vi "mules_date2string.vi"(6 "date slash?":bool, 7 "time":timestamp, 8 "time colon?":bool, 9 "seconds?":bool, 10 "log_time":bool, 11 "now?":bool=TRUE) -> (1 "time_string":string, 2 "mm/dd/yyyy":string, 3 "date_time_string":string)   [LabVIEW 2013]
doc: "Da formato a los datos de fecha y hora."
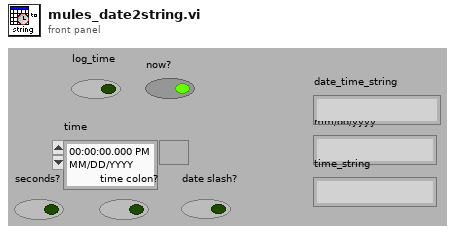
[diagram p1: front panel]
types:
  T1 = typedef "LVDateTimeRec.ctl" = cluster{"fractional second":dbl, "second":i32, "minute":i32, "hour":i32, "day of month":i32, "month":i32, "year":i32, "day of week":i32, "day of year":i32, "DST":i32}
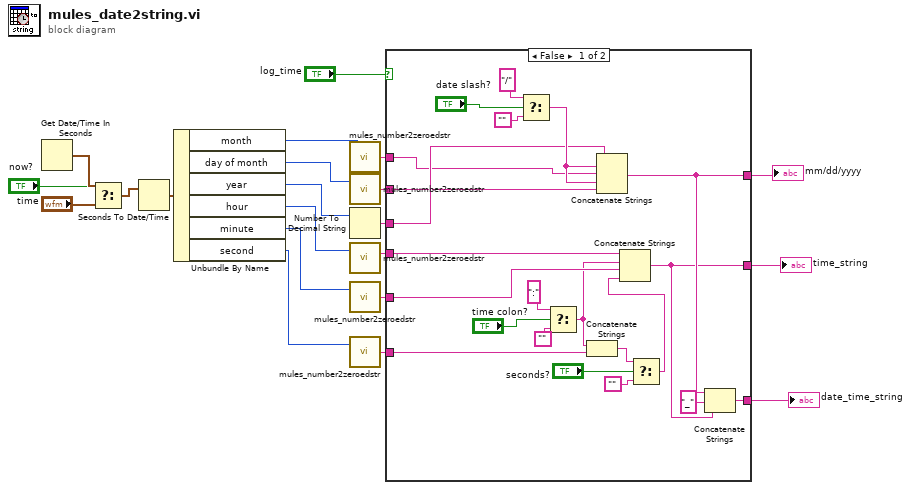
[diagram p0: block diagram]
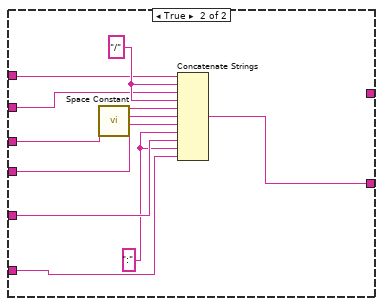
[diagram p2: hidden frame]
diagram:
  n1 = Get Date/Time In Seconds() -> (seconds since 1Jan1904=w3:timestamp)
  n2 = Select(t=w3, s="now?", f="time") -> (s? t:f=w2:timestamp)
  n3 = Seconds To Date/Time(time stamp (now)=w2) -> (date time rec=w21:T1)  [unwired: 1 out]
  n4 = Unbundle By Name(w21) -> ("month"=w10:i32, "day of month"=w9:i32, "year"=w8:i32, "hour"=w7:i32, "minute"=w6:i32, "second"=w5:i32)
  n5 = call "mules_number2zeroedstr.vi"("number"=w10) -> ("string"=w20:string)  [unwired: 1 in]
  n6 = call "mules_number2zeroedstr.vi"("number"=w9) -> ("string"=w19:string)  [unwired: 1 in]
  n7 = Number To Decimal String(number=w8) -> (decimal integer string=w18:string)  [unwired: 1 out]
  n8 = call "mules_number2zeroedstr.vi"("number"=w7) -> ("string"=w17:string)  [unwired: 1 in]
  n9 = call "mules_number2zeroedstr.vi"("number"=w6) -> ("string"=w16:string)  [unwired: 1 in]
  n10 = call "mules_number2zeroedstr.vi"("number"=w5) -> ("string"=w15:string)  [unwired: 1 in]
  n11 = case shown="False" "log_time" {
    tunnel: w20 -> [w23 w45]
    tunnel: w19 -> [w22 w44]
    tunnel: w18 -> [w24 w52]
    tunnel: w17 -> [w36 w50]
    tunnel: w16 -> [w35 w49]
    tunnel: w15 -> [w34 w47]
    tunnel: [w28 _] -> w13
    tunnel: [w25 w46] -> w12
    tunnel: [w26 _] -> w11
    frame False {
      n12 = Select(t="/", s="date slash?", f="") -> (s? t:f=w41:string)
      n13 = Select(t=":", s="time colon?", f="") -> (s? t:f=w33:string)
      n14 = Concatenate Strings(w33, w34) -> (w32:string)
      n15 = Concatenate Strings(w24, w41, w23, w41, w22) -> (w28:string)
      n16 = Select(t=w32, s="seconds?", f="") -> (s? t:f=w29:string)
      n17 = Concatenate Strings(w36, w33, w35, w29) -> (w25:string)
      n18 = Concatenate Strings(w28, "_", w25) -> (w26:string)
    }
    frame True {
      w48 = ":"
      w53 = "/"
      n19 = call <vilib>:"Space Constant.vi"() -> ("String"=w51:string)
      n20 = Concatenate Strings(w45, w53, w44, w53, w52, w51, w50, w48, w49, w48, w47) -> (w46:string)
    }
  }
  "mm/dd/yyyy" <- w13
  "time_string" <- w12
  "date_time_string" <- w11
